vi "Cumulate Time.vi"(8 "error in":errorcluster, 11 "Chronometer in":refnum<class "Chronometer.lvclass">) -> (0 "error out":errorcluster, 3 "Chronometer out":refnum<class "Chronometer.lvclass">)   [LabVIEW 2023, in "Chronometer.lvlib" / "Chronometer.lvclass"]
uses:
  Chronometer.lvclass
  Chronometer.lvclass/Chronometer.ctl
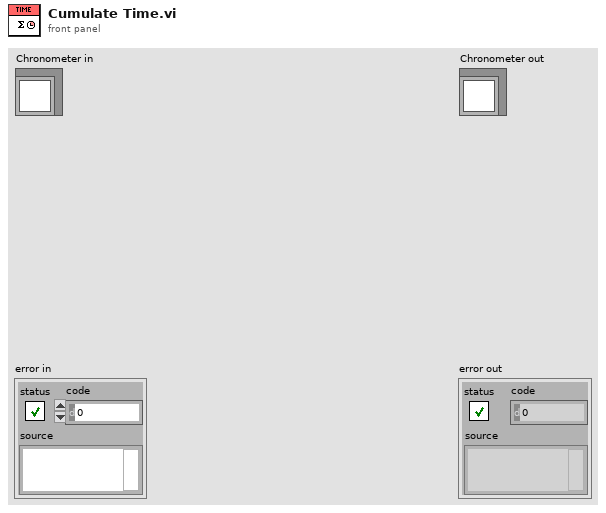
[diagram p1: front panel]
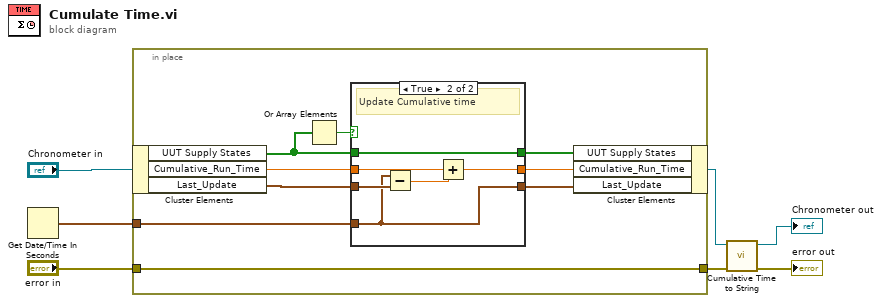
[diagram p0: block diagram]
diagram:
  n1 = Get Date/Time In Seconds() -> (seconds since 1Jan1904=w5:timestamp)
  n2 = in-place {
    in-place-border: "error in" -> [w8]
    in-place-border: w5 -> [w13]
    in-place-border: [w8] -> w3
    n3 = in-place-cluster #1("Chronometer in") -> ("UUT Supply States"=w15:bool[], "Cumulative_Run_Time"=w12:dbl, "Last_Update"=w10:timestamp)
    n4 = Or Array Elements(Boolean array=w15) -> (logical OR=w16:bool)
    n5 = case shown="True" w16 {
      tunnel: w15 -> [w19 w25]
      tunnel: [w19 w25] -> w14
      tunnel: w13 -> [w17 w20]
      tunnel: w12 -> [w18 w22]
      tunnel: [w18 w21] -> w11
      tunnel: w10 -> [_ w24]
      tunnel: [w17 w20] -> w9
      frame False {
        # "Update Last Update Time"
      }
      frame True {
        # "Update Cumulative time"
        n6 = Subtract(x=w20, y=w24) -> (x-y=w23:dbl)
        n7 = Add(x=w22, y=w23) -> (x+y=w21:dbl)
      }
    }
    n8 = in-place-cluster #1("UUT Supply States"=w14, "Cumulative_Run_Time"=w11, "Last_Update"=w9) -> (w4:refnum<class "Chronometer.lvclass">)
  }
  n9 = call "Cumulative Time to String.vi"("error in"=w3, "Chronometer in"=w4) -> ("error out"=→"error out":errorcluster, "Chronometer out"=→"Chronometer out":refnum<class "Chronometer.lvclass">)  [unwired: 8 in]
